vi "Flatten Load & Unload.vi"(8 "Error In":errorcluster, 11 "Load & Unload.lvclass":refnum<class "Load & Unload.lvclass">) -> (0 "Error Out":errorcluster, 3 "String":string)   [LabVIEW 2020, in "lv_icon.lvlib"]
uses:
  resource/plugins/lv_icon.lvlib
  Classes/Load_Unload/Load & Unload.lvclass
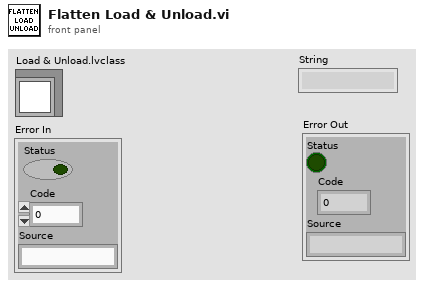
[diagram p1: front panel]
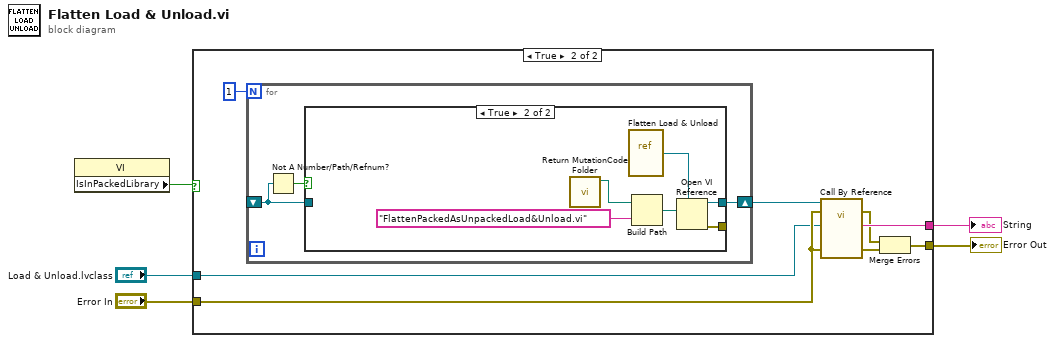
[diagram p0: block diagram]
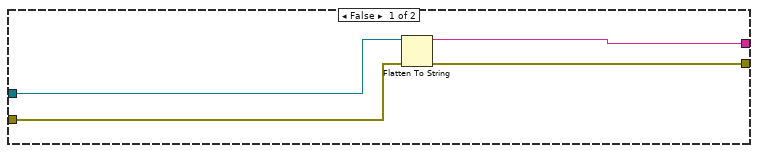
[diagram p2: hidden frame]
diagram:
  n1 = property class="VI"() -> ("IsInPackedLibrary"=w1:bool)  [unwired: 2 in, 2 out]
  n2 = case shown="True" w1 {
    tunnel: [w8 w17] -> w5
    tunnel: [w9 w16] -> w4
    tunnel: "Error In" -> [w7 w15]
    tunnel: "Load & Unload.lvclass" -> [w6 w10]
    frame False {
      n3 = Flatten To String(anything=w6, error in (no error)=w7) -> (data string=w8:string, error out=w9:errorcluster)  [unwired: 2 in, 1 out]
    }
    frame True {
      n4 = for {
        N: 1 -> [_]
        shift-right: [w18] -> w13
        shift-left: _ -> [w19]
        n5 = Not A Number/Path/Refnum?(number/path/refnum=w19) -> (NaN/Path/Refnum?=w20:bool)
        n6 = case shown="True" w20 {
          tunnel: [w21 w25] -> w18
          tunnel: w19 -> [w21 _]
          tunnel: [_ w23] -> _
          frame False {
          }
          frame True {
            n7 = call "Return MutationCode Folder.vi"() -> ("Base Path Mutation Code"=w24:path)  [unwired: 11 in]
            n8 = vi-ref "Flatten Load & Unload.vi"() -> (w22:refnum<vi>)
            n9 = Build Path(base path=w24, name or relative path="FlattenPackedAsUnpackedLoad&Unload.vi") -> (appended path=w26:path)
            n10 = Open VI Reference(type specifier VI Refnum (for type only)=w22, vi path=w26) -> (vi reference=w25:refnum<vi>, error out=w23:errorcluster)  [unwired: 4 in]
          }
        }
      }
      n11 = call-by-ref "?"(reference=w13, error in=w15, "Error In"=w15, "Load & Unload.lvclass"=w10) -> (error out=w11:errorcluster, "Error Out"=w12:errorcluster, "String"=w17:string)  [unwired: 8 in, 1 out]
      n12 = Merge Errors(w11, w12) -> (w16:errorcluster)
    }
  }
  "String" <- w5
  "Error Out" <- w4
